vi "PicoScope6000aProcessStreamingDataTriggerInfo.vi"(2 "enabled array":i16[](array[numeric])=[1, 0, 0, 0, 0, 0, 0, 0, 0, 0], 7 "tPicoStreamingDataTriggerInfo In":T1 {"autoStop_" step=1; "triggered_" step=1}, 9 "C Array for Struture Data In":u16[][](array[numeric]), 11 "error in":errorcluster) -> (8 "C Array for Struture Data Out":u16[][](array[numeric]), 10 "tPicoStreamingDataTriggerInfo":T1, 15 "error out":errorcluster)   [LabVIEW 2010]
doc: "This VIcan be used for one or two functions-\n-Converts a cluster defined for C struture defined to 2D array to pass to a C shared library function.\n-Converts a 2D array returned from a C shared library functionas an array of clusters representing the C struture"
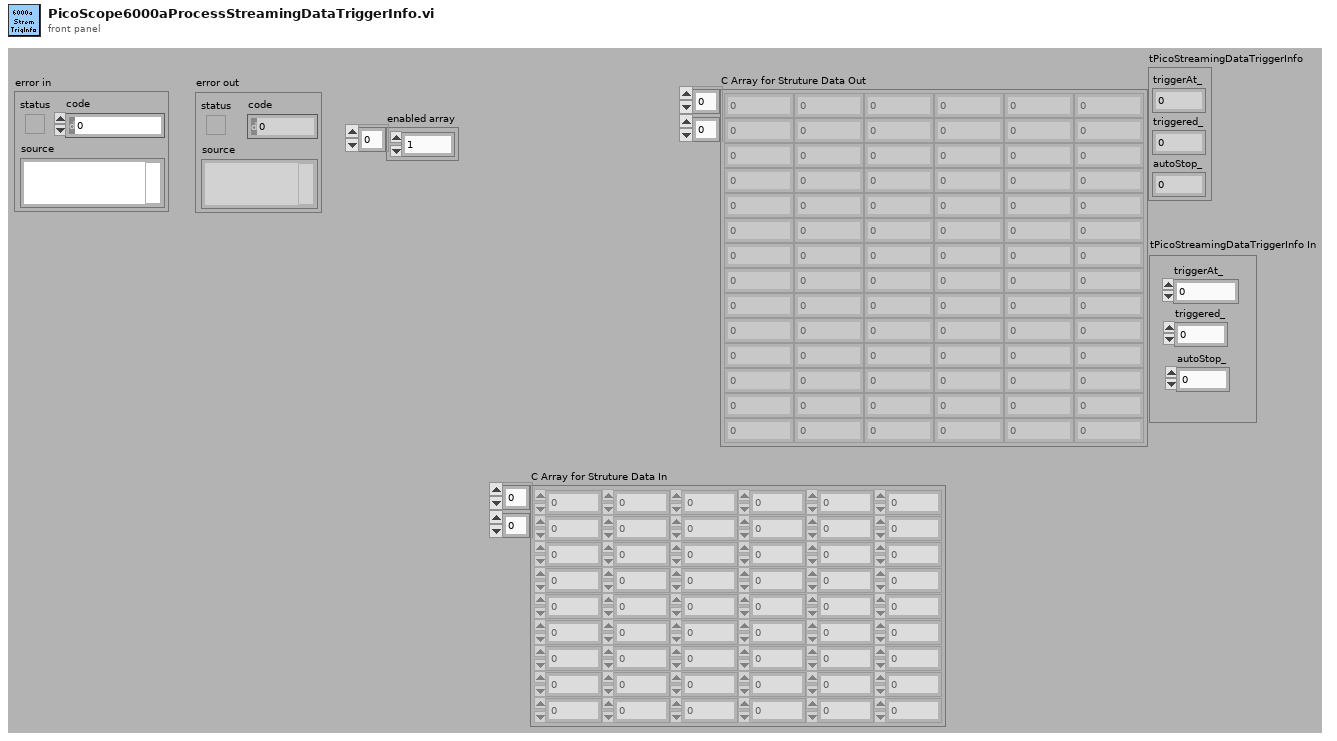
[diagram p1: front panel]
types:
  T1 = cluster{"triggerAt_":u64, "triggered_":i16, "autoStop_":i16}
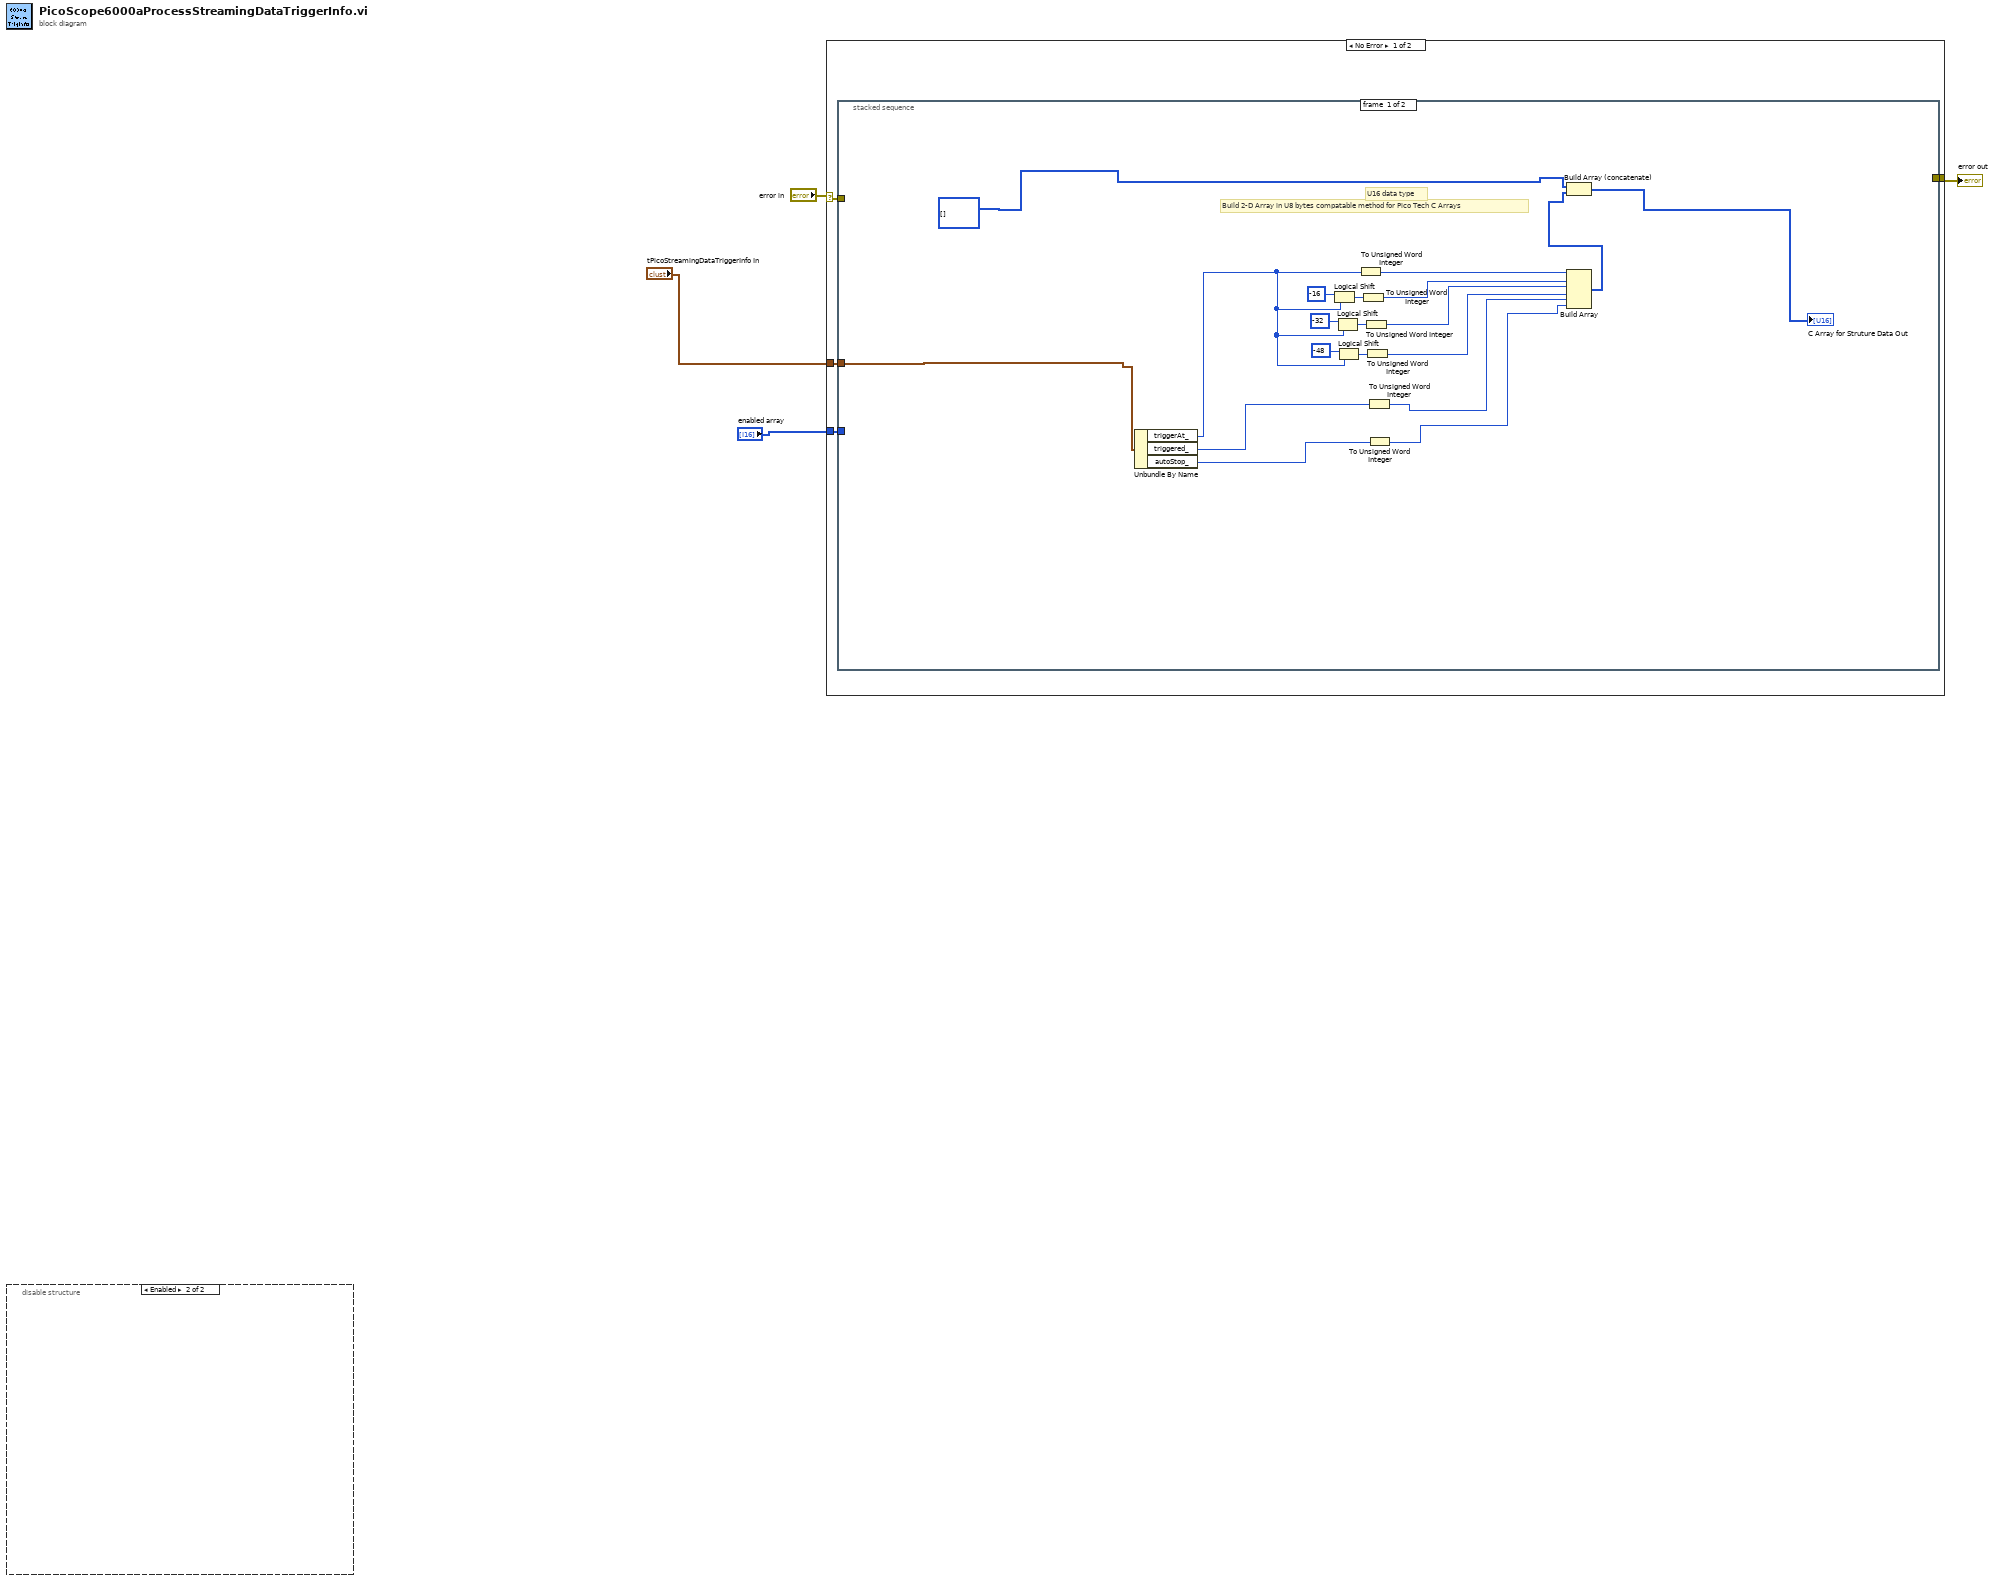
[diagram p0: block diagram]
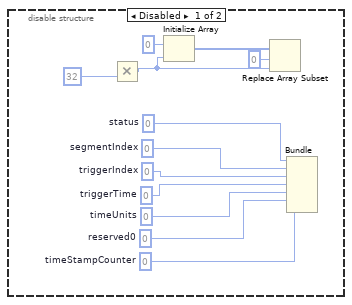
[diagram p2: hidden frame]
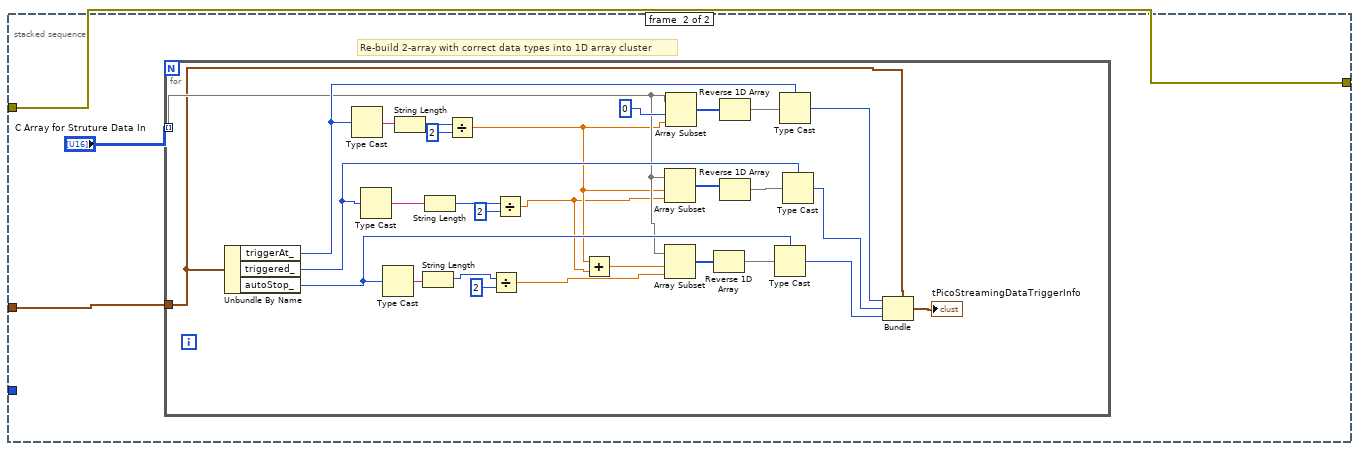
[diagram p3: hidden frame]
diagram:
  n1 = disable-structure shown="Enabled" {
    frame Disabled {
      w12 = u64 0  # timeStampCounter
      w10 = i16 0  # reserved0
      w11 = i16 0  # timeUnits
      w13 = i64 0  # triggerTime
      w14 = u32 0  # triggerIndex
      w15 = u32 0  # segmentIndex
      w16 = u32 0  # status
      n2 = Multiply(y=u32 32) -> (x*y=w8:u32)  [unwired: 1 in]
      n3 = Initialize Array(u8 0 ("element"), w8) -> (w9:u8[])
      n4 = Replace Array Subset(array=w9, new element=w8, index=0) -> ()  [unwired: 1 out]
      n5 = Bundle("status"=w16, "segmentIndex"=w15, "triggerIndex"=w14, "triggerTime"=w13, "timeUnits"=w11, "reserved0"=w10, "timeStampCounter"=w12) -> ()  [unwired: 1 in, 1 out]
    }
    frame Enabled {
    }
  }
  n6 = case shown="No Error" "error in" {
    selector: "error in" -> [w20 w72]
    tunnel: [w19 w72] -> w3
    tunnel: "tPicoStreamingDataTriggerInfo In" -> [w18 _]
    tunnel: "enabled array" -> [w17 _]
    frame No Error {
      n7 = stacked-sequence {
        tunnel: w20 -> [_ w42]
        tunnel: [_ w42] -> w19
        tunnel: w18 -> [w38 w41]
        tunnel: w17 -> [_ _]
        frame #0 {
          # "U16 data type"
          # "Build 2-D Array in U8 bytes compatable method for Pico Tech C Arrays"
          n8 = Unbundle By Name(w38) -> ("triggerAt_"=w27:u64, "triggered_"=w35:i16, "autoStop_"=w22:i16)
          n9 = Logical Shift(y=i16 -16, x=w27) -> (x << y=w30:u64)
          n10 = Logical Shift(y=i16 -32, x=w27) -> (x << y=w29:u64)
          n11 = Logical Shift(y=i16 -48, x=w27) -> (x << y=w28:u64)
          n12 = To Unsigned Word Integer(number=w27) -> (unsigned 16bit integer=w23:u16)
          n13 = To Unsigned Word Integer(number=w30) -> (unsigned 16bit integer=w24:u16)
          n14 = To Unsigned Word Integer(number=w29) -> (unsigned 16bit integer=w25:u16)
          n15 = To Unsigned Word Integer(number=w28) -> (unsigned 16bit integer=w26:u16)
          n16 = To Unsigned Word Integer(number=w35) -> (unsigned 16bit integer=w36:u16)
          n17 = To Unsigned Word Integer(number=w22) -> (unsigned 16bit integer=w21:u16)
          n18 = Build Array(w23, w24, w25, w26, w36, w21) -> (w34:u16[])
          n19 = Build Array (concatenate)(u16[][] [], w34) -> (→"C Array for Struture Data Out":u16[][])
        }
        frame #1 {
          # "Re-build 2-array with correct data types into 1D array cluster"
          n20 = for {
            tunnel: "C Array for Struture Data In" -> [w55] mode=indexing
            tunnel: w41 -> [w44]
            n21 = Unbundle By Name(w44) -> ("triggerAt_"=w58:u64, "triggered_"=w57:i16, "autoStop_"=w56:i16)
            n22 = Type Cast(x=w58) -> (*(type *) &x=w54:string)  [unwired: 1 in]
            n23 = Type Cast(x=w57) -> (*(type *) &x=w63:string)  [unwired: 1 in]
            n24 = Type Cast(x=w56) -> (*(type *) &x=w62:string)  [unwired: 1 in]
            n25 = String Length(string=w54) -> (length=w53:i32)
            n26 = String Length(string=w62) -> (length=w46:i32)
            n27 = String Length(string=w63) -> (length=w47:i32)
            n28 = Divide(x=w53, y=2) -> (x/y=w51:dbl)
            n29 = Divide(x=w46, y=2) -> (x/y=w45:dbl)
            n30 = Divide(x=w47, y=2) -> (x/y=w48:dbl)
            n31 = Add(x=w51, y=w48) -> (x+y=w60:dbl)
            n32 = Array Subset(array=w55, index=w51, length=w48) -> (w70:u16[])
            n33 = Array Subset(array=w55, index=w60, length=w45) -> (w65:u16[])
            n34 = Array Subset(array=w55, index=0, length=w51) -> (w68:u16[])
            n35 = Reverse 1D Array(array=w65) -> (reversed array=w66:u16[])
            n36 = Reverse 1D Array(array=w68) -> (reversed array=w67:u16[])
            n37 = Reverse 1D Array(array=w70) -> (reversed array=w69:u16[])
            n38 = Type Cast(type=w56, x=w66) -> (*(type *) &x=w71:i16)
            n39 = Type Cast(type=w58, x=w67) -> (*(type *) &x=w59:u64)
            n40 = Type Cast(type=w57, x=w69) -> (*(type *) &x=w64:i16)
            n41 = Bundle(cluster=w44, "triggerAt_"=w59, "triggered_"=w64, "autoStop_"=w71) -> (→"tPicoStreamingDataTriggerInfo":T1)
          }
        }
      }
    }
    frame Error {
    }
  }
  "error out" <- w3
